vi "Offset Widget Transaction Lists.vi"(7 "Offset Type":T5, 8 "error in (no error)":errorcluster, 9 "Coordinate Space":bool caption="Coord", 10 "Rigid Connection":bool, 11 "Number of\nLBCBs":T6) -> (0 "error out":errorcluster, 2 "Transactions":T2[](array[typedef]))   [LabVIEW 2009]
uses:
  Data Access Objects/Application/Number Of LBCBs.ctl
  Offset Types.ctl
  Global Data/Transactions/Dataset Transaction Id.ctl
  Global Data/Transactions/Dataset Source.ctl
  Global Data/Transactions/Dataset Type.ctl
  Apps/Yes No Button.ctl
panel:
  in  "Cartesian Types":T1[](array[typedef])=[enum."Displacement Command", enum."Displacement", enum."Force"]
  in  "Actuator Types":T1[](array[typedef])=[enum."Actuator Command", enum."LVDT", enum."Load Cell"]
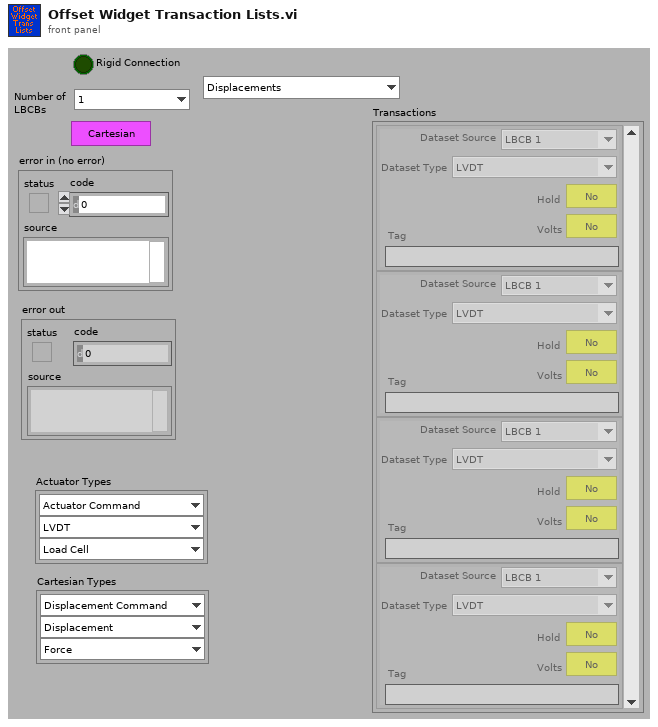
[diagram p1: front panel]
types:
  T1 = typedef "Dataset Type.ctl" = enum16{"LVDT", "Load Cell", "Actuator Command", "Servo Error", "Displacement Command", "Displacement", "Force"}
  T2 = typedef "Dataset Transaction Id.ctl" = cluster{"Dataset Source":T3, "Dataset Type":T1, "Hold":T4, "Volts":T4, "Tag":string}
  T3 = typedef "Dataset Source.ctl" = enum16{"LBCB 1", "LBCB 2", "Combined", "External Sensors"}
  T4 = typedef "Yes No Button.ctl" = bool
  T5 = typedef "Offset Types.ctl" = enum16{"Displacements", "Forces", "External Sensors"}
  T6 = typedef "Number Of LBCBs.ctl" = enum16{"1", "2"}
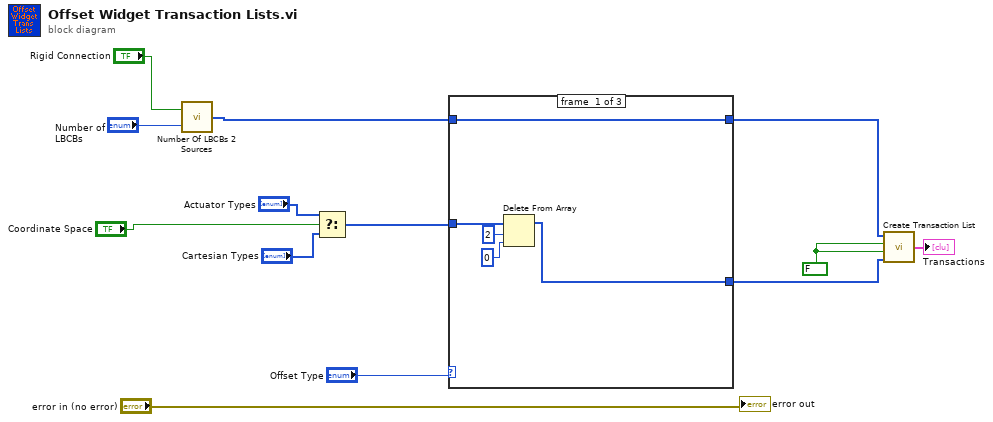
[diagram p0: block diagram]
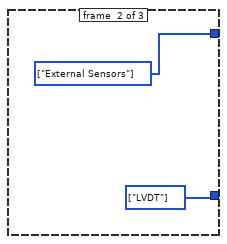
[diagram p2: hidden frame]
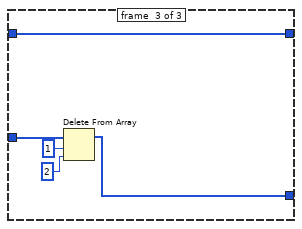
[diagram p3: hidden frame]
diagram:
  w13 = FALSE ("Include Volts")
  n1 = call "Number Of LBCBs 2 Sources.vi"("Number of LBCBs"="Number of\nLBCBs", "Combined LBCBs"="Rigid Connection") -> ("Sources"=w4:T3[])
  n2 = Select(t="Actuator Types", s="Coordinate Space", f="Cartesian Types") -> (s? t:f=w5:T1[])
  n3 = case shown="\"Displacements\"" "Offset Type" {
    tunnel: w5 -> [w18 _ w25]
    tunnel: w4 -> [w14 _ w21]
    tunnel: [w15 w20 w22] -> w3
    tunnel: [w14 w19 w21] -> w2
    frame #0 {
      n4 = Delete From Array(array=w18, length=2, index=0) -> (array with subset deleted=w15:T1[])  [unwired: 1 out]
    }
    frame #1 {
      w19 = T3[] [enum."External Sensors"] items=["LBCB 1", "LBCB 2", "Combined", "External Sensors"] ("Sources")
      w20 = T1[] [enum."LVDT"] items=["LVDT", "Load Cell", "Actuator Command", "Servo Error", "Displacement Command", "Displacement", "Force"] ("Types")
    }
    frame #2 {
      n5 = Delete From Array(array=w25, length=1, index=2) -> (array with subset deleted=w22:T1[])  [unwired: 1 out]
    }
  }
  n6 = call "Create Transaction List.vi"("Types"=w3, "Hold"=w13, "Volts"=w13, "Sources"=w2) -> ("Transactions"=→"Transactions":T2[])
  "error out" <- "error in (no error)"
